vi "2.vi"() -> ()   [LabVIEW 2015]
uses:
  <vilib>/measure/NI_MABase.lvlib
panel:
  in  "数值":dbl
  out "XY图":cluster{"Y":dbl[], "Y":dbl[]}(graph)
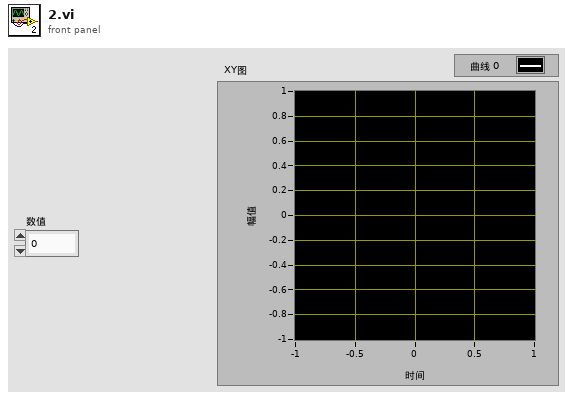
[diagram p1: front panel]
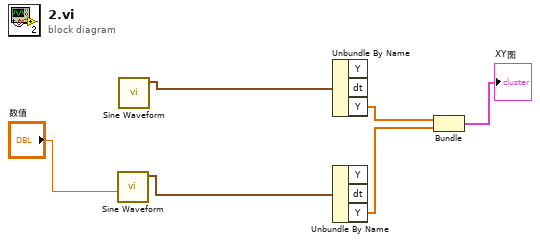
[diagram p0: block diagram]
diagram:
  n1 = call <vilib>:"Sine Waveform.vi"("phase"="数值") -> ("signal out"=w3:waveform(dbl))  [unwired: 9 in, 1 out]
  n2 = call <vilib>:"Sine Waveform.vi"() -> ("signal out"=w2:waveform(dbl))  [unwired: 10 in, 1 out]
  n3 = Unbundle By Name(w2) -> ("Y"=w6:dbl[])  [unwired: 2 out]
  n4 = Unbundle By Name(w3) -> ("Y"=w5:dbl[])  [unwired: 2 out]
  n5 = Bundle("Y"=w6, "Y"=w5) -> (→"XY图":cluster{"Y":dbl[], "Y":dbl[]})  [unwired: 1 in]
